vi "add cycle error graph.vi"(7 "Coords":T2, 8 "error in":errorcluster, 10 "DATA CLUSTER in":T1, 11 "CtlRef":refnum<vi>) -> (0 "error out":errorcluster, 2 "graph out":T3(array[cluster]))   [LabVIEW 2016]
uses:
  <vilib>/Utility/miscctls.llb/LVPoint32TypeDef.ctl
  controls/data control cluster.ctl
panel:
  out "Yerror 2":dbl[](array[numeric])
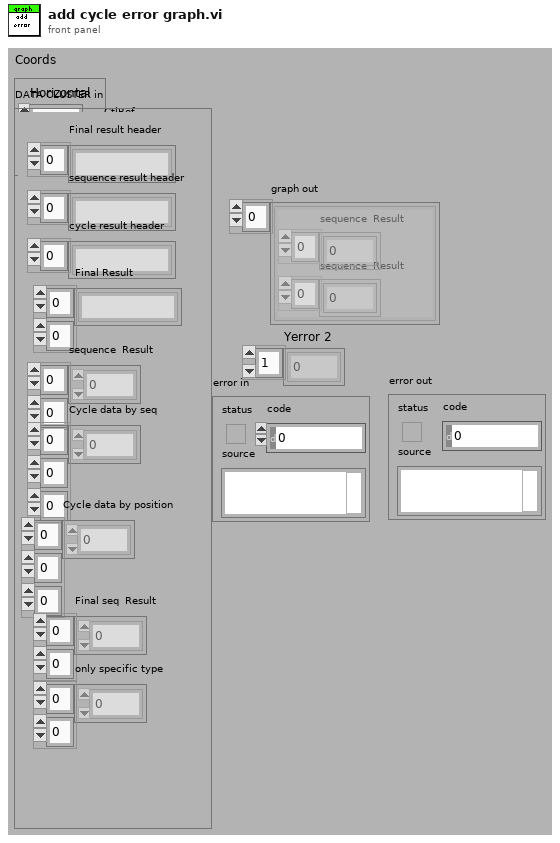
[diagram p1: front panel]
types:
  T1 = typedef "data control cluster.ctl" = cluster{"Final result header":string[], "sequence result header":string[], "cycle result header ":string[], "Final Result":string[][], "sequence  Result":dbl[][], "Cycle data by seq":dbl[][][], "Cycle data by position":dbl[][][], "Final seq  Result":dbl[][], "only specific type":dbl[][]}
  T2 = typedef "LVPoint32TypeDef.ctl" = cluster{"Horizontal":i32, "Vertical":i32}
  T3 = cluster{"sequence  Result":dbl[], "sequence  Result":dbl[]}[]
  T4 = cluster{"sequence  Result":dbl[], "sequence  Result":dbl[]}
  T5 = cluster{"Cycle data by seq":dbl[], "Cycle data by seq":dbl[]}
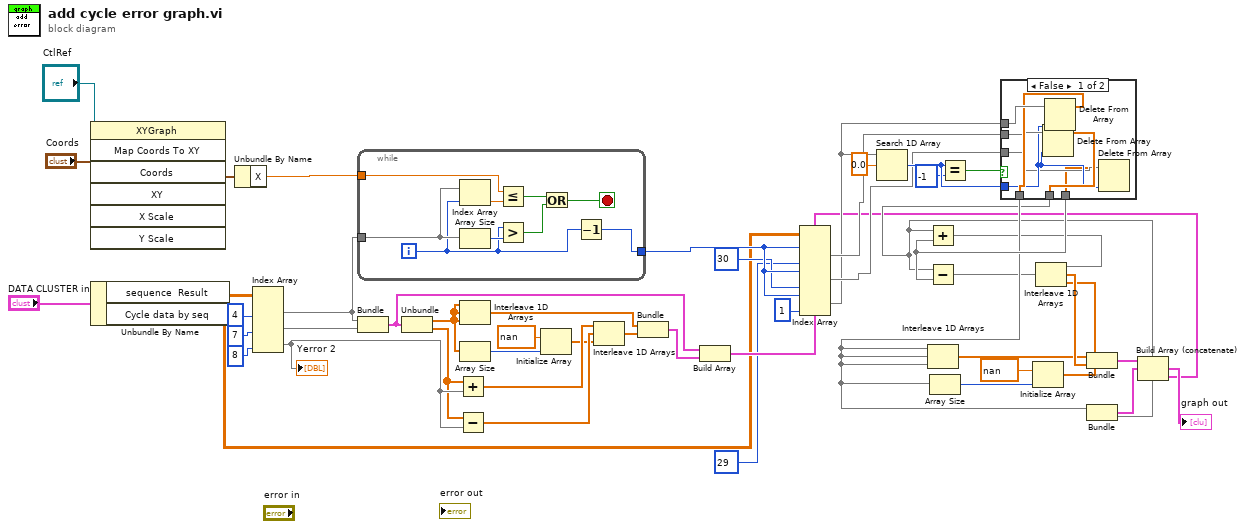
[diagram p0: block diagram]
diagram:
  n1 = invoke class="XYGraph" method="Map Coords To XY"(reference="CtlRef", "Coords"="Coords") -> ("XY"=w22:cluster{"X":dbl, "Y":dbl})  [unwired: 5 in, 6 out]
  n2 = Unbundle By Name("DATA CLUSTER in") -> ("sequence  Result"=w5:dbl[][], "Cycle data by seq"=w1:dbl[][][])
  n3 = Unbundle By Name(w22) -> ("X"=w23:dbl)
  n4 = Index Array(array=w5, index (col) #1=4 ("disabled index (col)"), index (col) #2=7 ("index (col)"), index (col) #3=8 ("index (col)")) -> (element #1=w24:dbl[], element #2=w10:dbl[], element #3=w9:dbl[])  [unwired: 3 in]
  "Yerror 2" <- w9
  n5 = while {
    tunnel: w23 -> [w54]
    tunnel: w24 -> [w58]
    tunnel: [w50] -> w28
    i -> [w51]
    stop <- w55 stop-if-true
    n6 = Index Array(array=w58, index=w51) -> (element=w53:dbl)
    n7 = Array Size(array=w58) -> (size(s)=w57:i32)
    n8 = Less Or Equal?(x=w54, y=w53) -> (x <= y?=w52:bool)
    n9 = Greater?(x=w51, y=w57) -> (0:w56:bool)
    n10 = Or(x=w52, y=w56) -> (x .or. y?=w55:bool)
    n11 = Decrement(x=w51) -> (x-1=w50:i32)
  }
  n12 = Bundle("sequence  Result"=w24, "sequence  Result"=w10) -> (w11:T4)  [unwired: 1 in]
  n13 = Unbundle(w11) -> ("sequence  Result"=w2:dbl[], "sequence  Result"=w3:dbl[])
  n14 = Add(x=w3, y=w9) -> (x+y=w17:dbl[])
  n15 = Subtract(x=w3, y=w9) -> (x-y=w16:dbl[])
  n16 = Interleave 1D Arrays(w2, w2, w2) -> (w18:dbl[])
  n17 = Array Size(array=w2) -> (size(s)=w15:i32)
  n18 = Initialize Array(nan ("element"), w15) -> (w14:dbl[])
  n19 = Interleave 1D Arrays(w17, w16, w14) -> (w19:dbl[])
  n20 = Bundle(w18, w19) -> (w12:cluster{dbl[], dbl[]})  [unwired: 1 in]
  n21 = Build Array(w11, w12) -> (w38:T3)
  n22 = Index Array(array=w1, index (dim 0) #1=w28, index (dim 2) #1=29 ("disabled index (col)"), index (dim 0) #2=w28, index (dim 2) #2=30 ("index (col)"), index (dim 0) #3=w28, index (dim 2) #3=1 ("index (col)")) -> (element #1=w44:dbl[], element #2=w47:dbl[], element #3=w43:dbl[])  [unwired: 3 in]
  n23 = Search 1D Array(1D array=w43, element=0.0) -> (index of element=w49:i32)  [unwired: 1 in]
  n24 = Equal?(x=w49, y=-1) -> (x = y?=w42:bool)
  n25 = case shown="False" w42 {
    tunnel: w44 -> [w63 w68]
    tunnel: w43 -> [w65 w67]
    tunnel: [w62 w68] -> w45
    tunnel: [w64 w67] -> w46
    tunnel: w47 -> [w60 w66]
    tunnel: [w59 w66] -> w48
    tunnel: w49 -> [w61 _]
    frame False {
      n26 = Delete From Array(array=w63, index=w61) -> (array with subset deleted=w62:dbl[])  [unwired: 1 in, 1 out]
      n27 = Delete From Array(array=w65, index=w61) -> (array with subset deleted=w64:dbl[])  [unwired: 1 in, 1 out]
      n28 = Delete From Array(array=w60, index=w61) -> (array with subset deleted=w59:dbl[])  [unwired: 1 in, 1 out]
    }
    frame True {
    }
  }
  n29 = Add(x=w45, y=w48) -> (x+y=w29:dbl[])
  n30 = Subtract(x=w45, y=w48) -> (x-y=w30:dbl[])
  n31 = Interleave 1D Arrays(w46, w46, w46) -> (w32:dbl[])
  n32 = Array Size(array=w46) -> (size(s)=w31:i32)
  n33 = Initialize Array(nan ("element"), w31) -> (w34:dbl[])
  n34 = Interleave 1D Arrays(w29, w30, w34) -> (w35:dbl[])
  n35 = Bundle(w32, w35) -> (w36:cluster{dbl[], dbl[]})  [unwired: 1 in]
  n36 = Bundle("Cycle data by seq"=w46, "Cycle data by seq"=w45) -> (w37:T5)  [unwired: 1 in]
  n37 = Build Array (concatenate)(w36, w37, w38) -> (→"graph out":T3)
